vi "Get-receiver-channels.vi"(8 "error in (no error)":errorcluster, 10 "Receivers":string[](array[string]), 11 "ModComm in":T1) -> (0 "error out":errorcluster, 2 "Receiver channels":refnum<queue>[](array[refnum]), 3 "ModComm out":T1)   [LabVIEW 2013, in "Server.lvlib" / "Server.lvclass"]
uses:
  Server.lvclass
  Object-reference.ctl
  Messages/Sources/Message.lvclass
  Supported-module-types.ctl
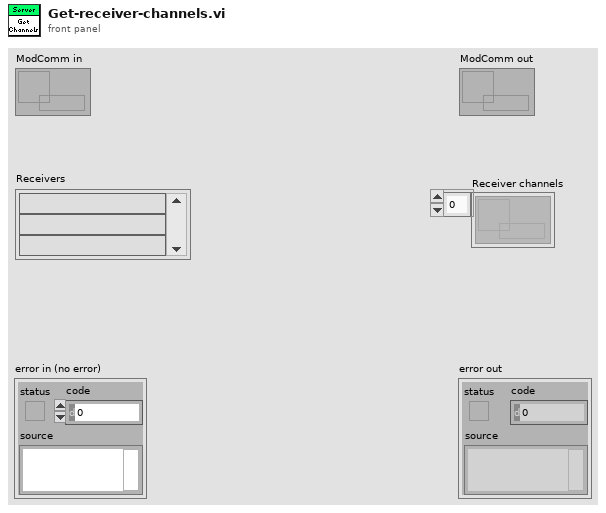
[diagram p1: front panel]
types:
  T1 = typedef "Server.lvlib/Server.lvclass/Object-reference.ctl" = refnum<data-value>
  T2 = typedef "Server.lvlib/Server.lvclass/Supported-module-types.ctl" = enum16{"Server", "All", "BeamControl", "PowderDeposition", "StrategyParser", "CameraVision", "MaterialCharacterization", "StatusMonitor", "SLMSimulation", "LaserCharacterization"}
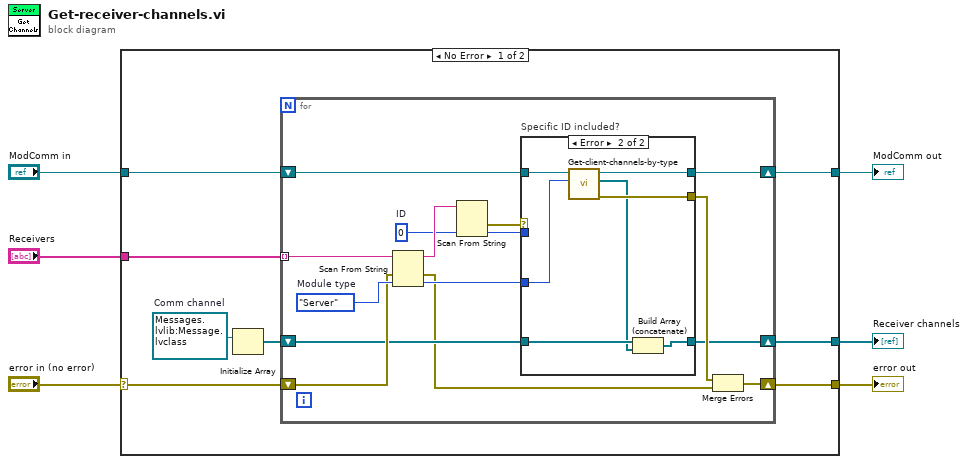
[diagram p0: block diagram]
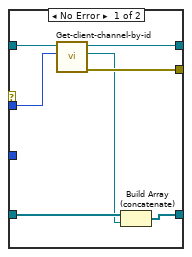
[diagram p2: hidden frame]
diagram:
  n1 = case shown="No Error" "error in (no error)" {
    selector: "error in (no error)" -> [w11 w45]
    tunnel: [w7 w45] -> w5
    tunnel: [w13 w44] -> w3
    tunnel: "ModComm in" -> [w14 w44]
    tunnel: "Receivers" -> [w12 _]
    tunnel: [w8 _] -> w1
    frame No Error {
      w10 = refnum<queue> refnum  # Comm channel
      n2 = Initialize Array(w10) -> (w9:refnum<queue>[])  [unwired: 1 in]
      n3 = for {
        tunnel: w12 -> [w29] mode=indexing
        shift-right: [w18] -> w7
        shift-left: w11 -> [w27]
        shift-right: [w15] -> w8
        shift-left: w9 -> [w19]
        shift-right: [w20] -> w13
        shift-left: w14 -> [w21]
        w25 = 0  # ID
        w28 = Supported-module-types."Server"  # Module type
        n4 = Scan From String(input string=w29, error in=w27, default 1=w28) -> (remaining string=w26:string, error out=w17:errorcluster, output 1=w22:T2)  [unwired: 2 in, 1 out]
        n5 = Scan From String(input string=w26, default 1=w25) -> (error out=w24:errorcluster, output 1=w23:i32)  [unwired: 3 in, 2 out]
        n6 = case "Specific ID included?" shown="Error" w24 {
          tunnel: w23 -> [w34 _]
          tunnel: w22 -> [_ w43]
          tunnel: w21 -> [w36 w42]
          tunnel: [w35 w41] -> w20
          tunnel: [w33 w40] -> w16
          tunnel: w19 -> [w32 w39]
          tunnel: [w30 w38] -> w15
          frame No Error {
            n7 = call "Get-client-channel-by-id.vi"("Client ID"=w34, "ModComm in"=w36) -> ("error out"=w33:errorcluster, "Client channel"=w31:refnum<queue>, "ModComm out"=w35:T1)  [unwired: 7 in]
            n8 = Build Array (concatenate)(w32, w31) -> (w30:refnum<queue>[])
          }
          frame Error {
            n9 = call "Get-client-channels-by-type.vi"("Module type"=w43, "ModComm in"=w42) -> ("error out"=w40:errorcluster, "Client channels"=w37:refnum<queue>[], "ModComm out"=w41:T1)  [unwired: 7 in]
            n10 = Build Array (concatenate)(w39, w37) -> (w38:refnum<queue>[])
          }
        }
        n11 = Merge Errors(w16, w17) -> (w18:errorcluster)
      }
    }
    frame Error {
    }
  }
  "error out" <- w5
  "ModComm out" <- w3
  "Receiver channels" <- w1
